vi "Close Logging.vi"(8 "error in":errorcluster) -> (0 "error out":errorcluster)   [LabVIEW 2020, in "hse-logger.lvlib"]
doc: "Close the logger and clean up all registered handler.\n\n____\nHAMPEL SOFTWARE ENGINEERING v2.0.6 (2021-04-15 11:38)"
uses:
  hse-logger.lvlib
  FGV Actions.ctl
  Logger/Logger.lvclass
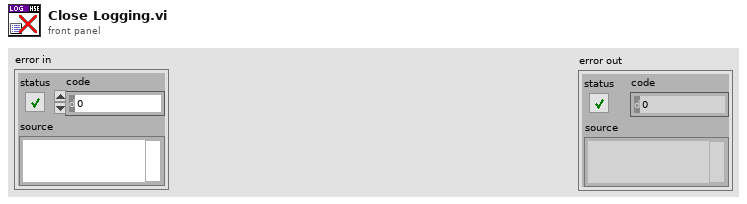
[diagram p1: front panel]
types:
  T1 = typedef "hse-logger.lvlib/FGV Actions.ctl" = enum16{"Set", "Get"}
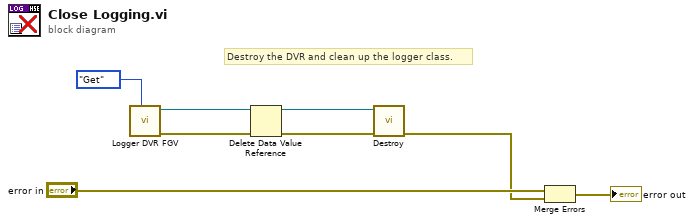
[diagram p0: block diagram]
diagram:
  # "Destroy the DVR and clean up the logger class."
  n1 = call "Logger DVR FGV.vi"("FGV Actions"=FGV_Actions."Get") -> ("error out"=w3:errorcluster, "Logger DVR"=w4:refnum<data-value>)  [unwired: 9 in]
  n2 = Delete Data Value Reference(data value reference=w4, error in=w3) -> (data value=w1:refnum<class "Logger.lvclass">, error out=w2:errorcluster)
  n3 = call-dynamic "Destroy.vi"("error in"=w2, "Logger in"=w1) -> ("error out"=w5:errorcluster)  [unwired: 8 in, 1 out]
  n4 = Merge Errors("error in", w5) -> (→"error out":errorcluster)
